vi "DRIVE_RESET_ENCODERS.vi"(10 "argv":string[](array[string]), 11 "args":u8) -> ()   [LabVIEW 2011]
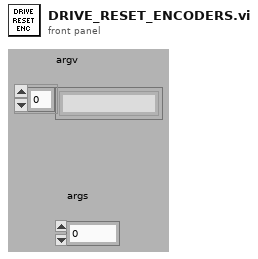
[diagram p1: front panel]
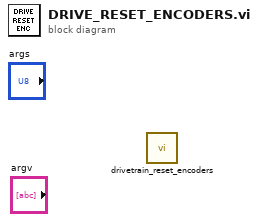
[diagram p0: block diagram]
diagram:
  n1 = call "drivetrain_reset_encoders.vi"() -> ()  [unwired: 9 in, 3 out]
